vi "New Event.vi"(11 "Channel Data In":T1) -> (3 "Channel Data":T1, 5 "Event Reg":refnum<event-registration>)   [LabVIEW 2022 SP3, in "Flex.lvlib"]
uses:
  Flex.lvlib
  Channel Data.ctl
  Event Data.ctl
  Element.ctl
  Writer Data.ctl
  Queue Data.ctl
  Element Info.ctl
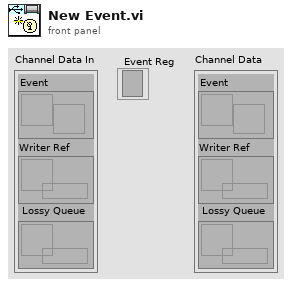
[diagram p1: front panel]
types:
  T1 = typedef "Flex.lvlib/Channel Data.ctl" = cluster{"Event":refnum<user-event>, "Writer Ref":refnum<data-value>, "Lossy Queue":refnum<queue>}
  T2 = typedef "Flex.lvlib/Writer Data.ctl" = cluster{"Lossless":refnum<queue>[], "Events":bool, "Lossy":bool}
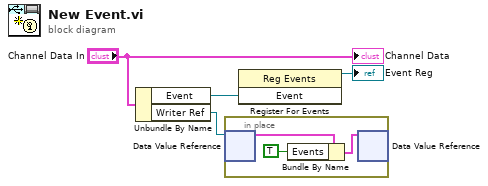
[diagram p0: block diagram]
diagram:
  n1 = Unbundle By Name("Channel Data In") -> ("Event"=w2:refnum<user-event>, "Writer Ref"=w1:refnum<data-value>)
  n2 = in-place {
    n3 = in-place-dvr #1(w1) -> (w7:T2)  [unwired: 1 out]
    n4 = Bundle By Name(cluster=w7, "Events"=TRUE) -> (w5:T2)
    n5 = in-place-dvr #1(w5) -> ()  [unwired: 2 out]
  }
  n6 = register-events(w2) -> (reference out=→"Event Reg":refnum<event-registration>)  [unwired: 2 in, 1 out]
  "Channel Data" <- "Channel Data In"
